vi "Subtract.vi"(1 "x":sgl, 2 "y":sgl, 4 "Subtractor0":refnum<class "Subtractor0.lvclass">) -> (6 "x-y":sgl)   [LabVIEW 2017, in "Subtractor0.lvclass"]
uses:
  Subtractor0.lvclass
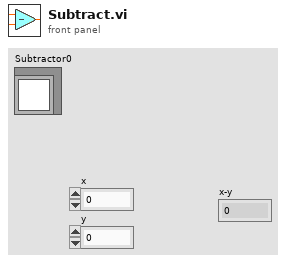
[diagram p1: front panel]
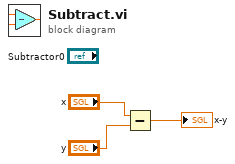
[diagram p0: block diagram]
diagram:
  n1 = Subtract(x="x", y="y") -> (x-y=→"x-y":sgl)
